vi "Calculate Base Array.vi"(8 "error in (no error)":errorcluster, 10 "2D Feather Datatype.lvclass in":refnum<class "2D Feather Datatype.lvclass">, 11 "Plot Representation In":T1) -> (0 "error out":errorcluster, 2 "2D Feather Datatype.lvclass out":refnum<class "2D Feather Datatype.lvclass">, 3 "Plot Representation Out":T1)   [LabVIEW 2017, in "2D Feather Datatype.lvclass"]
uses:
  <vilib>/Math Plots/2D Math Plots/2D Feather/2D Feather Datatype/2D Feather Datatype.lvclass
  <vilib>/Math Plots/2D Math Plots/2D Plot/2D Plot/Typedef/Plot Representation.ctl
  <vilib>/Math Plots/2D Math Plots/2D Plot/2D Plot/Typedef/Range Cluster.ctl
  <vilib>/Math Plots/2D Math Plots/2D Feather/2D Feather Datatype/2D Feather Datatype.lvclass/2D Feather Datatype.ctl
  <vilib>/Math Plots/2D Math Plots/2D Plot/2D Plot/2D Plot.lvclass
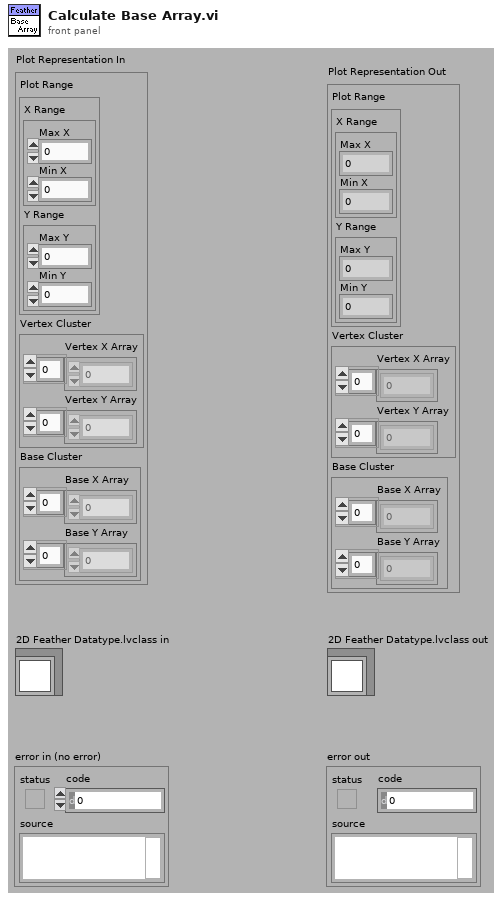
[diagram p1: front panel]
types:
  T1 = typedef "2D Plot.lvclass/Plot Representation.ctl" = cluster{"Plot Range":T2, "Vertex Cluster":cluster{"Vertex X Array":dbl[], "Vertex Y Array":dbl[]}, "Base Cluster":cluster{"Base X Array":dbl[], "Base Y Array":dbl[]}}
  T2 = typedef "2D Plot.lvclass/Range Cluster.ctl" = cluster{"X Range":cluster{"Max X":dbl, "Min X":dbl}, "Y Range":cluster{"Max Y":dbl, "Min Y":dbl}}
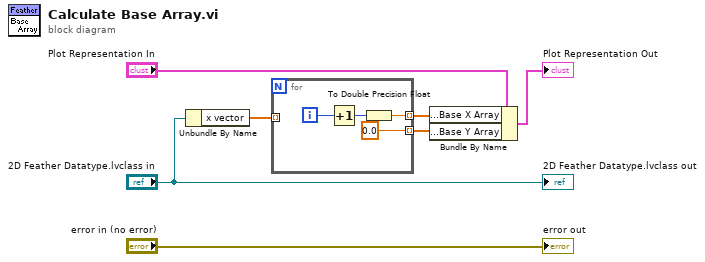
[diagram p0: block diagram]
diagram:
  n1 = Unbundle By Name("2D Feather Datatype.lvclass in") -> ("x vector"=w1:dbl[])
  n2 = for {
    tunnel: [0.0] -> w3 mode=indexing
    tunnel: [w8] -> w2 mode=indexing
    tunnel: w1 -> [_] mode=indexing
    i -> [w10]
    n3 = Increment(x=w10) -> (x+1=w9:i32)
    n4 = To Double Precision Float(number=w9) -> (double precision float=w8:dbl)
  }
  n5 = Bundle By Name(cluster="Plot Representation In", "Base Cluster.Base X Array"=w2, "Base Cluster.Base Y Array"=w3) -> (→"Plot Representation Out":T1)
  "2D Feather Datatype.lvclass out" <- "2D Feather Datatype.lvclass in"
  "error out" <- "error in (no error)"
